vi "Emballage_BDD_Creation_Certificat.vi"(8 "Error in":errorcluster caption="Error in (no error)", 11 "CODE BARRE du produit correspondant au certificat":string) -> (0 "Error out":errorcluster)   [LabVIEW 2020]
uses:
  Modules/FS/60_FS_Controles/60_FS_SetGet.ctl
panel:
  out "Chaîne":string
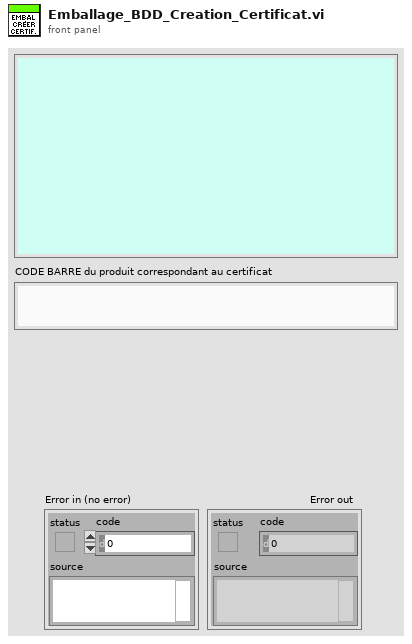
[diagram p1: front panel]
types:
  T1 = enum32{"Invalid", "Standard", "Closed", "Hidden", "Minimized", "Maximized"}
  T2 = typedef "60_FS_SetGet.ctl" = enum16{"set", "get"}
  T3 = typedef "Emballage_BDD_param_Produit.ctl" = cluster{"No_Valve_FAS":string, "suffixe":string, "designation":string, "indice_produit":string, "code_barre_fixe":string, "affiche_code_barre_client":string, "affiche_no_client":string, "Nb_vlve_par_carton":u16, "melange_des_lots_possible":string, "id_article":string, "Indice_Rev":string, "Famille":string, "date":string, "code_barre_fixe_Fin":string, "Longeur_No_Serie":string}
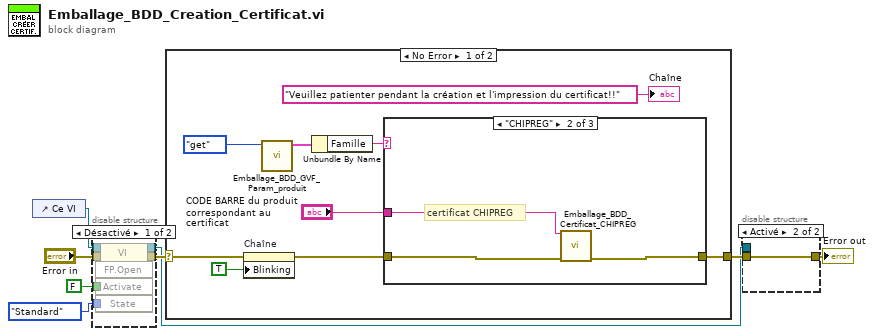
[diagram p0: block diagram]
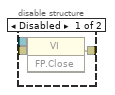
[diagram p2: hidden frame]
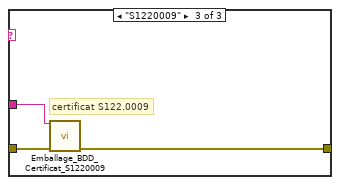
[diagram p5: hidden frame]
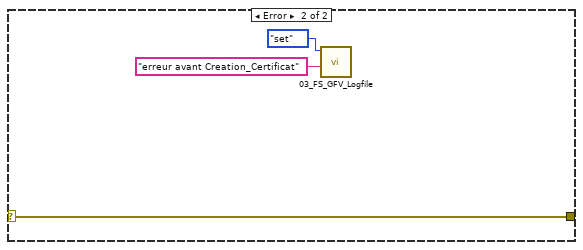
[diagram p6: hidden frame]
diagram:
  n1 = control-ref of="Ce VI"() -> (w5:refnum<vi>)
  n2 = disable-structure shown="Désactivé" {
    disable-tunnel: "Error in" -> [w14 w16]
    disable-tunnel: [w13 w16] -> w6
    disable-tunnel: w5 -> [w12 w15]
    disable-tunnel: FALSE ("Activer ?") -> [w11 _]
    disable-tunnel: T1."Standard" ("État") -> [w10 _]
    disable-tunnel: [w9 w15] -> w1
    frame Disabled {
      n3 = invoke class="VI" method="FP.Open"(reference=w12, error in=w14, "Activate"=w11, "State"=w10) -> (reference out=w9:refnum<vi>, error out=w13:errorcluster)  [unwired: 1 in, 3 out]
    }
    frame Enabled {
    }
  }
  n4 = case shown="No Error" w6 {
    selector: w6 -> [w20 w35]
    tunnel: [w23 w35] -> w7
    frame No Error {
      n5 = property on="Chaîne" class="Str"(error in=w20, "Blinking"=TRUE ("Clignotant")) -> (error out=w19:errorcluster)  [unwired: 1 in, 1 out]
      n6 = call "Emballage_BDD_GVF_Param_produit.vi"("Énum"=enum16{"set", "get"}."get") -> ("CLS_param_produit"=w24:T3)  [unwired: 7 in, 3 out]
      n7 = Unbundle By Name(w24) -> ("Famille"=w17:string)
      n8 = case shown="\"CHIPREG\"" w17 {
        tunnel: w19 -> [w26 w29 w31]
        tunnel: [w26 w28 w30] -> w23
        tunnel: "CODE BARRE du produit correspondant au certificat" -> [_ w27 w32]
        frame "", Default {
          # "Pas de certificat pour ce produit/famille"
        }
        frame "CHIPREG" {
          # "certificat CHIPREG"
          n9 = call "Emballage_BDD_Certificat_CHIPREG.vi"("CODE BARRE"=w27, "error in (no error)"=w29) -> ("error out"=w28:errorcluster)  [unwired: 12 in, 1 out]
        }
        frame "S1220009" {
          # "certificat S122.0009"
          n10 = call "Emballage_BDD_Certificat_S1220009.vi"("CODE BARRE"=w32, "error in (no error)"=w31) -> ("error out"=w30:errorcluster)  [unwired: 12 in, 1 out]
        }
      }
      "Chaîne" <- "Veuillez patienter pendant la création et l'impression du certificat!!" ("Chaîne")
    }
    frame Error {
      n11 = call "03_FS_GFV_Logfile.vi"("Chaîne"="erreur avant Creation_Certificat", "States"=60_FS_SetGet."set") -> ()  [unwired: 8 in, 2 out]
    }
  }
  n12 = disable-structure shown="Activé" {
    disable-tunnel: w7 -> [w38 w39]
    disable-tunnel: [w37 w39] -> w2
    disable-tunnel: w1 -> [w36 _]
    frame Disabled {
      n13 = invoke class="VI" method="FP.Close"(reference=w36, error in=w38) -> (error out=w37:errorcluster)  [unwired: 1 in, 2 out]
    }
    frame Enabled {
    }
  }
  "Error out" <- w2
